vi "ProcessFileFlow_Parse_EventRef.vi"(8 "error in (no error)":errorcluster, 11 "body":variant) -> (0 "error out":errorcluster, 3 "data":T1)   [LabVIEW 2017, in "FileFlow.lvlib"]
doc: "Converts the in-memory TDMS file and properties from the previous process in the Fileflow Script from variant data to its original cluster format."
uses:
  <vilib>/addons/InsightCM/Devices/Shared/Common/FileFlow/FileFlow.lvlib
  <vilib>/addons/InsightCM/Devices/Shared/Common/FileFlow/controls/data_eventRef.ctl
  <vilib>/addons/InsightCM/Devices/Shared/Common/DataEvent/controls/EventReference.ctl
  <vilib>/addons/InsightCM/Devices/Shared/Common/DataEvent/controls/Event.ctl
  <vilib>/addons/InsightCM/MessageBus/Base/controls/DataEvent.ctl
  <vilib>/addons/InsightCM/MessageBus/Base/controls/KeyValuePair.ctl
  <vilib>/addons/InsightCM/Devices/Shared/Common/DataEvent/controls/DataSet.ctl
  <vilib>/addons/InsightCM/MessageBus/Base/controls/DataSetMetadata.ctl
  <vilib>/addons/InsightCM/MessageBus/Base/controls/TrendPoint.ctl
  <vilib>/addons/InsightCM/MessageBus/Base/controls/TrendAlarmUpdate.ctl
  <vilib>/addons/InsightCM/MessageBus/Base/controls/TrendAlarmTransition.ctl
  <vilib>/addons/PointValueMap/controls/PointMap.ctl
  <vilib>/addons/PointValueMap/PointValueMap.lvlib
  <vilib>/addons/InsightCM/Devices/Shared/Common/DataEvent/DataEvent.lvlib
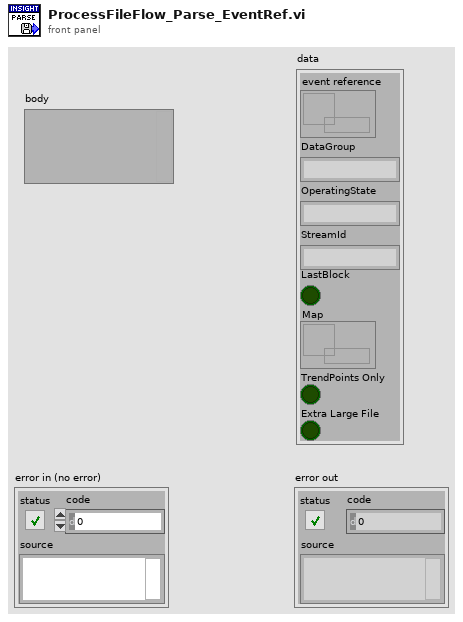
[diagram p1: front panel]
types:
  T1 = typedef "FileFlow.lvlib/data_eventRef.ctl" = cluster{"event reference":T2, "DataGroup":string, "OperatingState":string, "StreamId":string, "LastBlock":bool, "Map":T3, "TrendPoints Only":bool, "Extra Large File":bool}
  T2 = typedef "DataEvent.lvlib/EventReference.ctl" = refnum<data-value>
  T3 = typedef "PointValueMap.lvlib/PointMap.ctl" = refnum<data-value>
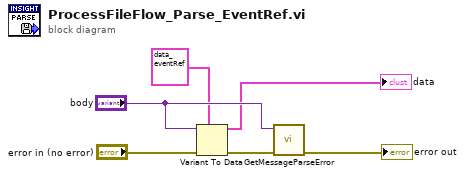
[diagram p0: block diagram]
diagram:
  n1 = Variant To Data(error in="error in (no error)", type=T1 {"event reference"=refnum, "DataGroup"="", "OperatingState"="", "StreamId"="", "LastBlock"=FALSE, "Map"=refnum, "TrendPoints Only"=FALSE, "Extra Large File"=FALSE} ("data"), Variant="body") -> (data=→"data":T1, error out=w6:errorcluster)
  n2 = call <vilib>:"GetMessageParseError.vi"("error in (no error)"=w6, "body"="body") -> ("error out"=→"error out":errorcluster)  [unwired: 7 in, 2 out]
